vi "niDTS BT INSTR RX Initiate.vi"(8 "error in (no error)":errorcluster, 9 "Result Index":i32=1, 10 "Driver Instance":i32=1, 11 "niDTS BT INSTR RX in":refnum<class "niDTS BT INSTR RX.lvclass">) -> (0 "error out":errorcluster, 3 "niDTS BT INSTR RX out":refnum<class "niDTS BT INSTR RX.lvclass">)   [LabVIEW 2015, in "niDTS BT.lvlib" / "niDTS BT INSTR RX.lvclass"]
uses:
  niDTS BT INSTR RX.lvclass
  niDTS BT INSTR RX.lvclass/niDTS BT INSTR RX.ctl
  RiviInstDriver/niRfsgBT/Objects/niRfsgBt.lvclass
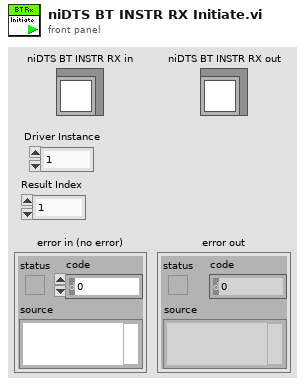
[diagram p1: front panel]
types:
  T1 = typedef "niRfsgBT.lvclass/niRfsgBT INC Handle.ctl" = refnum<data-value>
  T2 = typedef "niRfsgBt.lvclass/niRfsgBt INC Handle.ctl" = refnum<data-value>
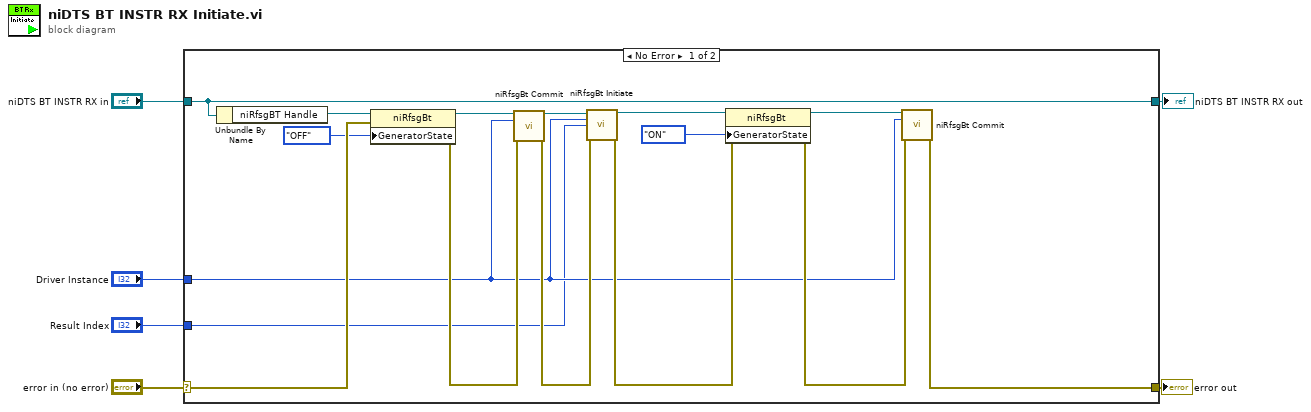
[diagram p0: block diagram]
diagram:
  n1 = case shown="No Error" "error in (no error)" {
    selector: "error in (no error)" -> [w18 w24]
    tunnel: [w22 w24] -> w5
    tunnel: [w9 w23] -> w3
    tunnel: "niDTS BT INSTR RX in" -> [w9 w23]
    tunnel: "Driver Instance" -> [w11 _]
    tunnel: "Result Index" -> [w10 _]
    frame No Error {
      n2 = Unbundle By Name(w9) -> ("niRfsgBT Handle"=w19:T1)
      n3 = property class="niRfsgBt"(reference=w19, error in=w18, "GeneratorState"=enum16{"OFF", "PENDING", "ON"}."OFF" ("SOURce:RFSG:BLUetooth:GeneratorState")) -> (reference out=w17:T1, error out=w16:errorcluster)
      n4 = call "niRfsgBt Commit.vi"("InstDriver Handle in"=w17, "Instance"=w11, "error in (no error)"=w16) -> ("InstDriver Handle out"=w15:T2, "error out"=w14:errorcluster)  [unwired: 11 in]
      n5 = call "niRfsgBt Initiate.vi"("InstDriver Handle in"=w15, "Driver Instance"=w11, "Result Instance"=w10, "error in (no error)"=w14) -> ("InstDriver Handle out"=w13:T1, "error out"=w12:errorcluster)  [unwired: 10 in]
      n6 = property class="niRfsgBt"(reference=w13, error in=w12, "GeneratorState"=enum16{"OFF", "PENDING", "ON"}."ON" ("SOURce:RFSG:BLUetooth:GeneratorState")) -> (reference out=w21:T1, error out=w20:errorcluster)
      n7 = call "niRfsgBt Commit.vi"("InstDriver Handle in"=w21, "Instance"=w11, "error in (no error)"=w20) -> ("error out"=w22:errorcluster)  [unwired: 11 in, 1 out]
    }
    frame Error {
    }
  }
  "error out" <- w5
  "niDTS BT INSTR RX out" <- w3
